vi "Main PXI4072.vi"() -> ()   [LabVIEW 2026]
uses:
  Drivers/PXI4072/Types/PXI4072 Settings.ctl
  <instrlib>/niDMM/nidmm.llb/niDMM Function.ctl
  <instrlib>/niDMM/nidmm.llb/niDMM Resolution in Digits.ctl
  App Types/Typedef/PXI4072 Runtime.ctl
  App Types/Typedef/PXI4072 Command Message.ctl
  App Types/Enums/PXI4072 Command.ctl
  App Types/Typedef/PXI4072 UI Update.ctl
  App Types/Enums/PXI4072 Instrument Triggered Events.ctl
  App Types/Enums/PXI4072 UI States.ctl
  App Types/References/PXI4072 All UI References.ctl
  App Types/References/PXI4072 Boolean UI References.ctl
  App Types/References/PXI4072 String UI References.ctl
  App Types/References/PXI4072 Numeric UI References.ctl
  App Types/References/PXI4072 Other UI Rerences.ctl
  Common/Types/Enum/Bench Modules.ctl
  <vilib>/event_ctls.llb/usereventprio.ctl
  App Types/Globals/PXI4072 UI Global Refs.vi
  UI/UI Manager/Actions/PXI4072 Set Refs.vi
  UI/UI Manager/Actions/PXI4072 Initialize.vi
  UI/UI Manager/Actions/PXI4072 Update UI Status.vi
  Drivers/PXI4072/PXI4072.lvlib
  Common/PXI_Common.lvlib
  Common/Types/Typedef/Log Message Levels.ctl
  Common/Types/Typedef/Log Message.ctl
panel:
  out "Measurement":dbl format="%.5f"
  in  "Measurement Settings":T1={"Function"=enum."DC Volts", "Resolution in Digits"=5.5, "Range"=10.0} {"Range" format="%.2f"; "Resolution in Digits" items=["3 1/2"=3.5, "4 1/2"=4.5, "5 1/2"=5.5, "6 1/2"=6.5, "7 1/2"=7.5]}
  in  "Apply Button":bool
  in  "Error":string
  out "Units":string
  in  "Reset Button":bool
  in  "Self Test Button":bool
  in  "Stop Button":bool
  in  "Continous Button":bool
  in  "Measure Button":bool
  in  "Status":string
  out "Connected?":bool
  in  "Disconnect Button":bool
  in  "Connect Button":bool
  in  "Resouce Name":refnum<k15> caption="Resource Name"
  out "error out":errorcluster
  in  "error in (no error)":errorcluster
  # "NI PXI-4072 DIGITAL MULTIMETER"
  # "MEASUREMENT SETUP"
  # "DEVICE"
  # "ACQUISITION"
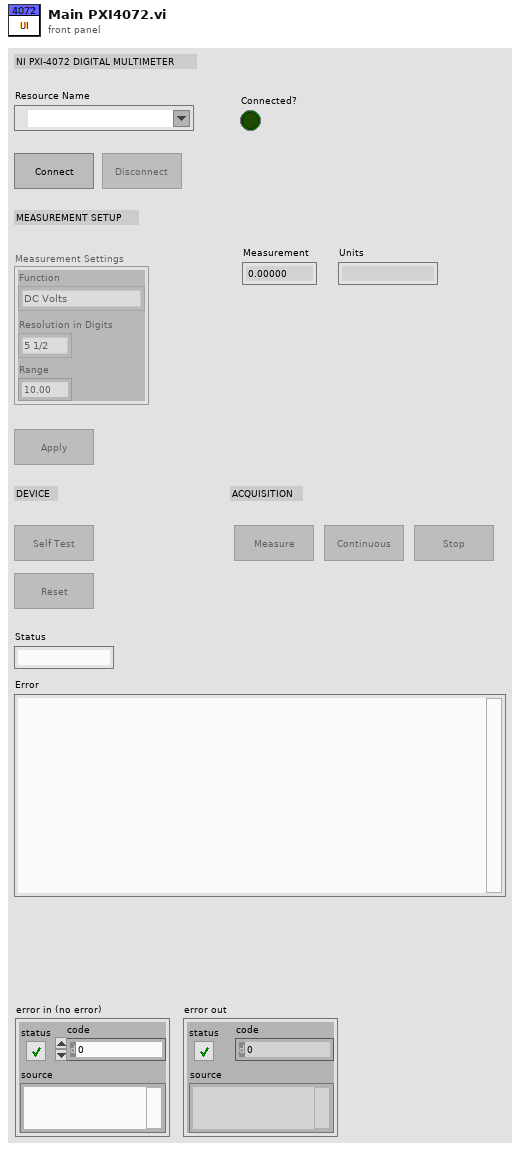
[diagram p1: front panel]
types:
  T1 = typedef "PXI4072.lvlib/PXI4072 Settings.ctl" = cluster{"Function":T2, "Resolution in Digits":T3, "Range":dbl}
  T2 = typedef "niDMM Function.ctl" = enum16{"DC Volts", "AC Volts", "DC Current", "AC Current", "2-wire Resistance", "4-wire Resistance", "Diode", "Frequency", "Period", "AC Volts DC Coupled", "Capacitance", "Inductance", "Temperature"}
  T3 = typedef "niDMM Resolution in Digits.ctl" = dbl
  T4 = typedef "PXI_Common.lvlib/Log Message.ctl" = cluster{"Timestamp":string, "Level":T5, "Instrument":T6, "Slot":string, "Code":i32, "Soruce":string, "Message":string}
  T5 = typedef "PXI_Common.lvlib/Log Message Levels.ctl" = enum16{"DEBUG", "INFO", "WARNING", "ERROR"}
  T6 = typedef "PXI_Common.lvlib/Bench Modules.ctl" = enum16{"Common", "PXI4072", "PXI6259", "PXI6224", "PXI4130", "PXI8431"}
  T7 = typedef "PXI4072 UI States.ctl" = enum16{"Get UI Refs", "UI Initialize", "Handle Events"}
  T8 = typedef "PXI4072 UI Update.ctl" = cluster{"Elements":cluster{"Event":T9, "Measurement":dbl, "Connected":bool, "Text":string, "Error":errorcluster}}
  T9 = typedef "PXI4072 Instrument Triggered Events.ctl" = enum16{"Measurement", "Connection", "Status", "Self Test", "Error"}
  T10 = typedef "PXI4072 Command Message.ctl" = cluster{"App Commands":T11, "Measurement Settings":T1}
  T11 = typedef "PXI4072 Command.ctl" = enum16{"Disconnect", "Initialize", "Configure", "Measure Single", "Reset", "Self Test", "Shutdown"}
  T12 = typedef "PXI4072 Runtime.ctl" = cluster{"Session Handle":refnum<k15>, "Measurement Settings":T1, "Connected":bool, "Last Measurement":dbl, "Last Error":errorcluster}
  T13 = typedef "PXI4072 All UI References.ctl" = cluster{"Boolean":T14, "String":T15, "Numeric":T16, "Other":T17}
  T14 = typedef "PXI4072 Boolean UI References.ctl" = cluster{"Connected?":refnum<vi>, "Reset Button":refnum<vi>, "Connect Button":refnum<vi>, "Apply Button":refnum<vi>, "Disconnect Button":refnum<vi>, "Measure Button":refnum<vi>, "Self Test Button":refnum<vi>, "Continous Button":refnum<vi>, "Stop Button":refnum<vi>}
  T15 = typedef "PXI4072 String UI References.ctl" = cluster{"Status":refnum<vi>, "Units":refnum<vi>, "Error":refnum<vi>}
  T16 = typedef "PXI4072 Numeric UI References.ctl" = cluster{"Measurement":refnum<vi>}
  T17 = typedef "PXI4072 Other UI Rerences.ctl" = cluster{"Resouce Name":refnum<vi>, "Measurement Settings":refnum<vi>}
  T18 = cluster{"Event":T9, "Measurement":dbl, "Connected":bool, "Text":string, "Error":errorcluster}
  T19 = typedef "usereventprio.ctl" = enum32{"high priority", "normal priority"}
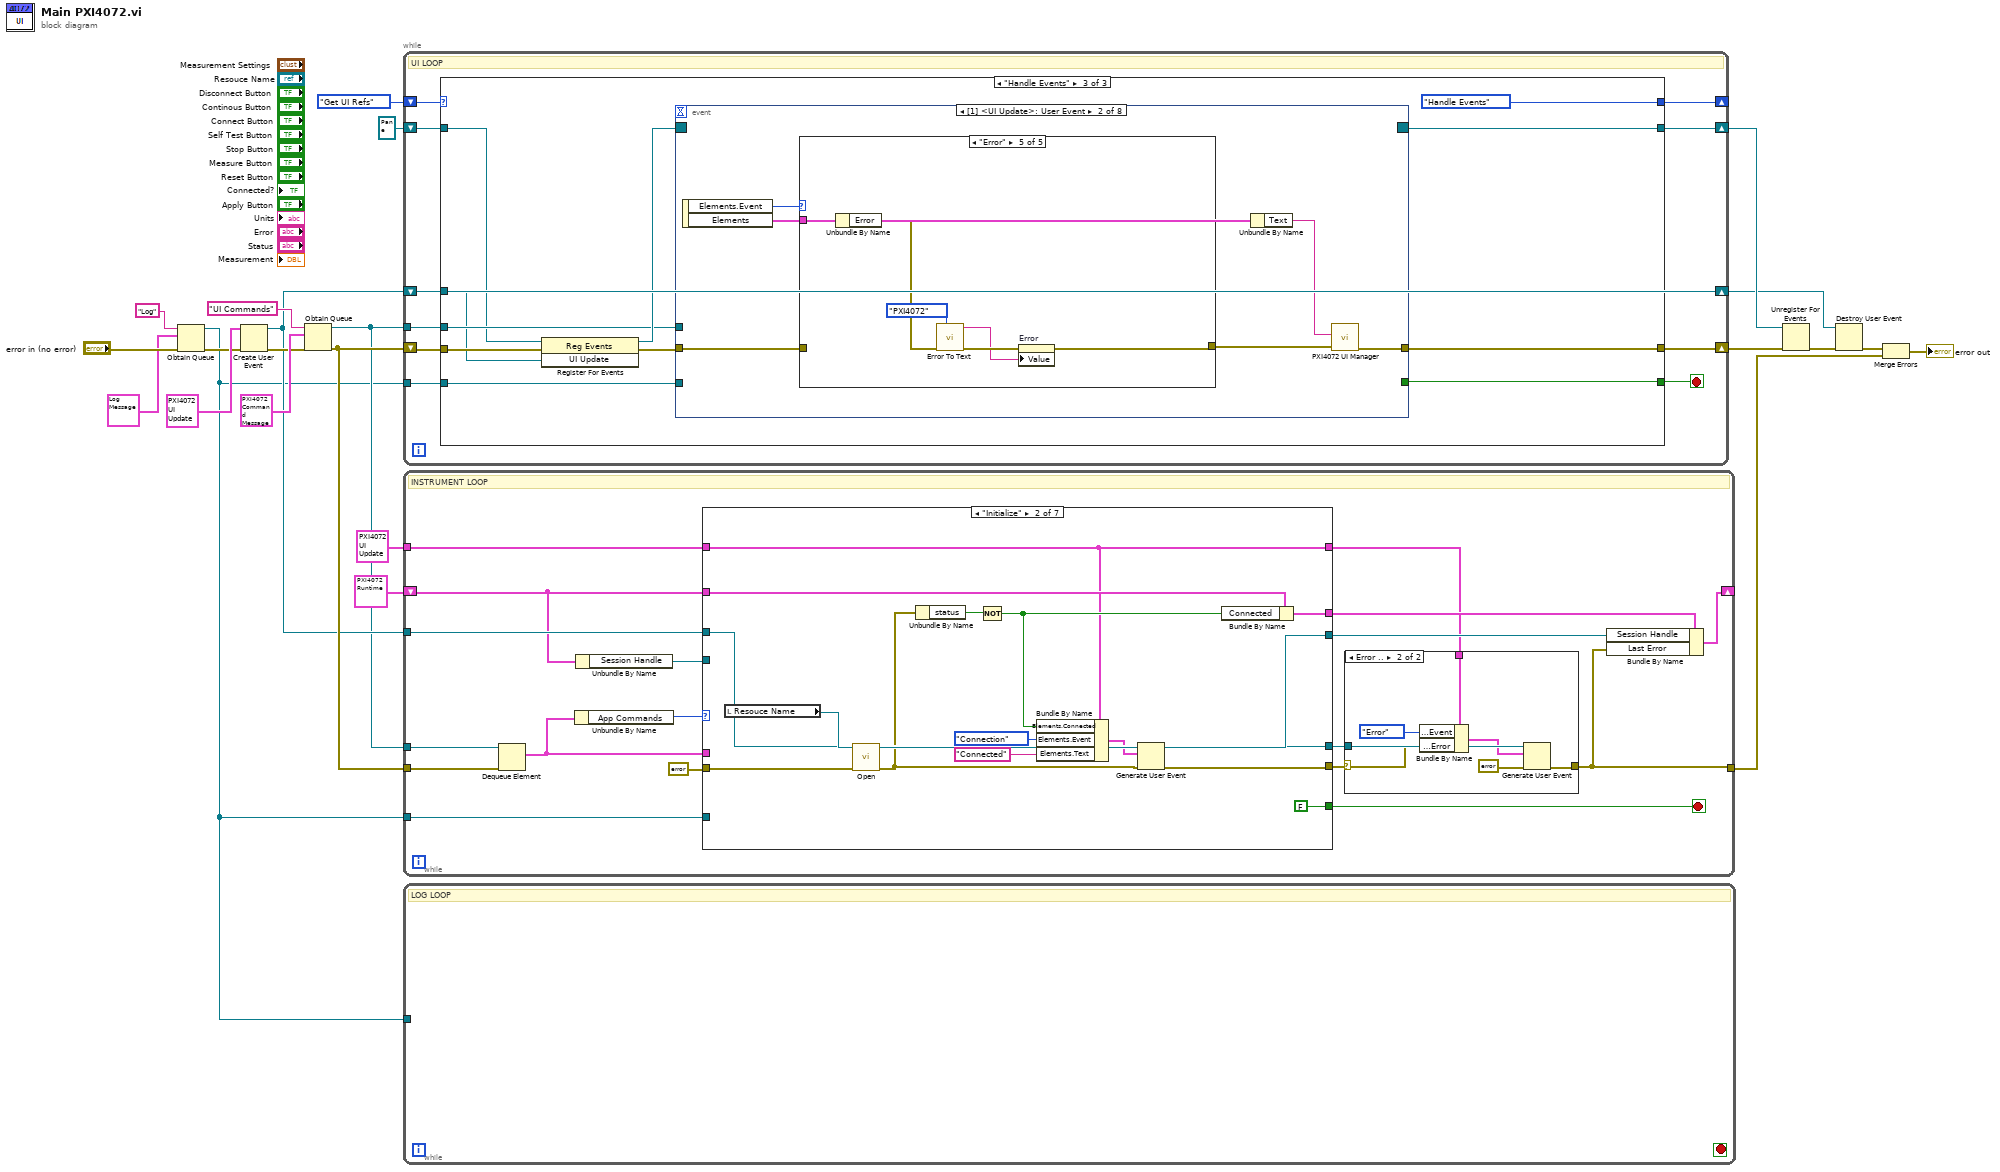
[diagram p0: block diagram]
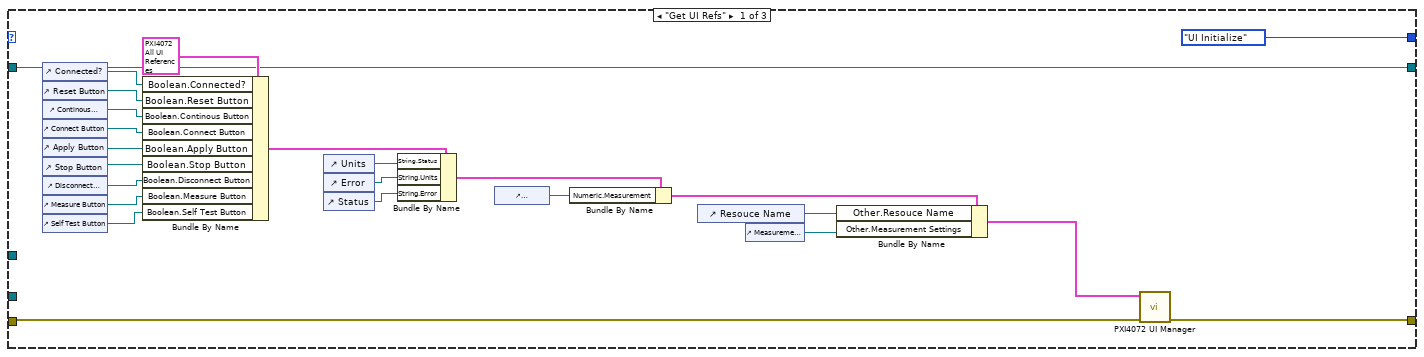
[diagram p2: hidden frame]
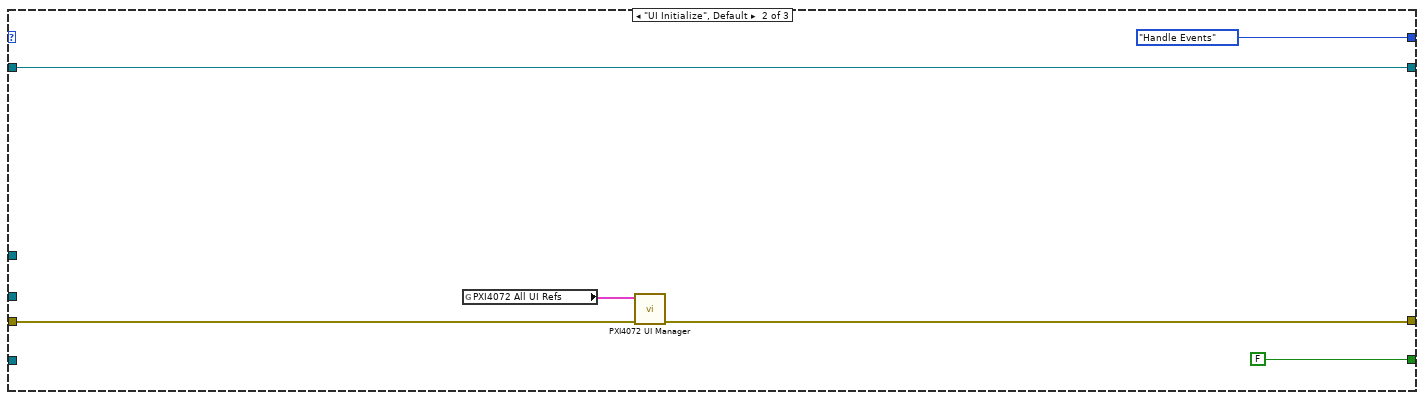
[diagram p3: hidden frame]
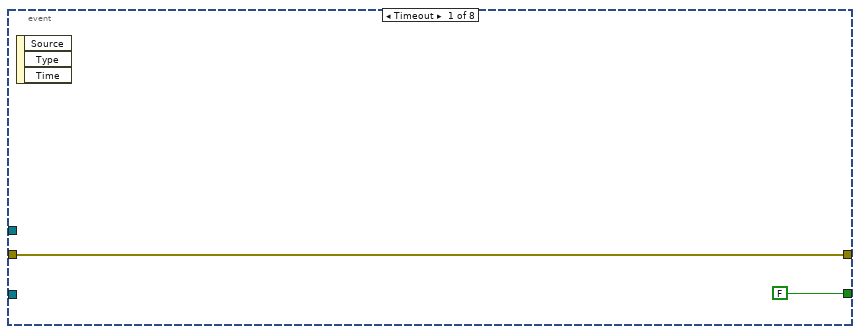
[diagram p4: hidden frame]
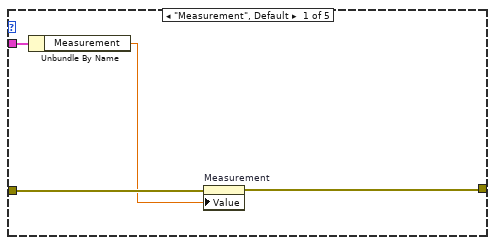
[diagram p5: hidden frame]
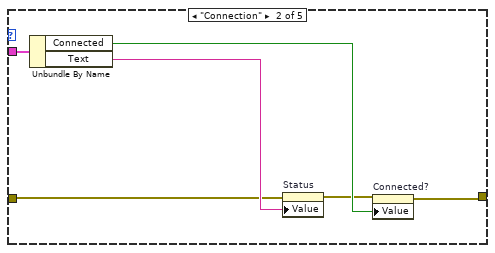
[diagram p6: hidden frame]
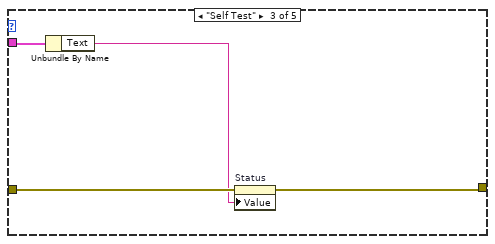
[diagram p7: hidden frame]
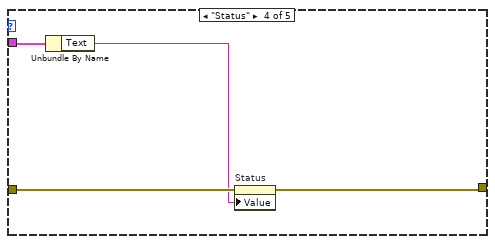
[diagram p8: hidden frame]
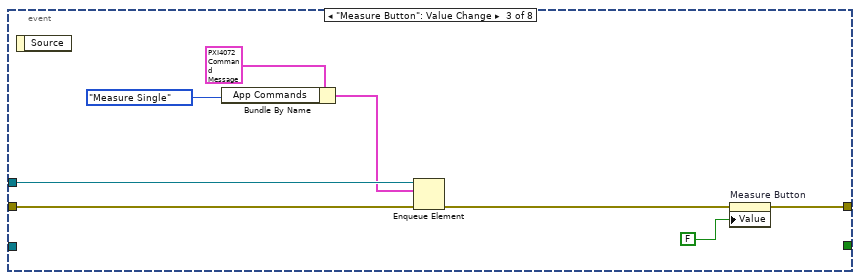
[diagram p9: hidden frame]
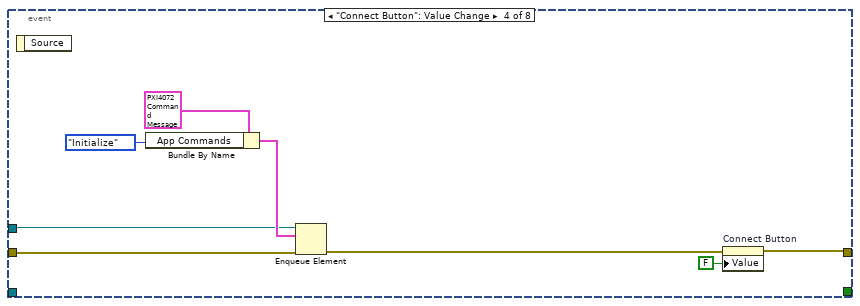
[diagram p10: hidden frame]
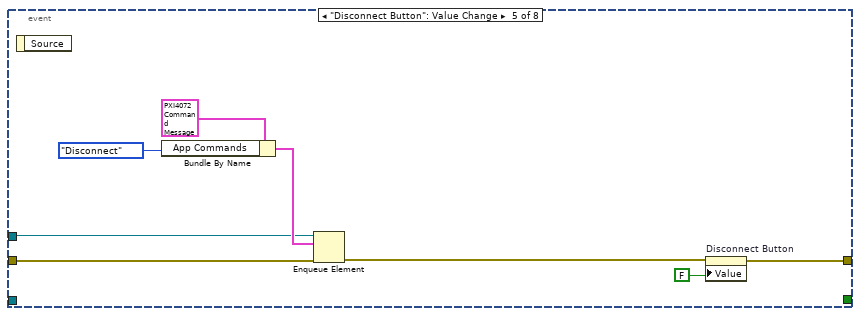
[diagram p11: hidden frame]
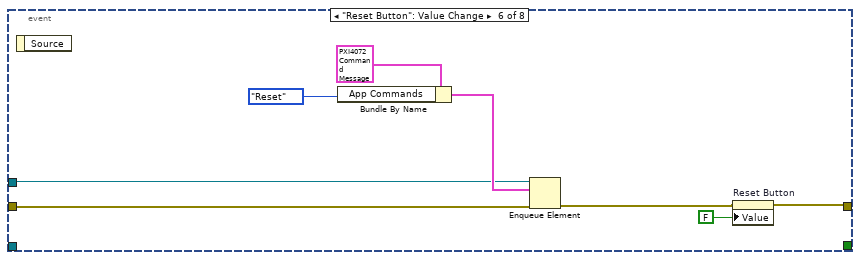
[diagram p12: hidden frame]
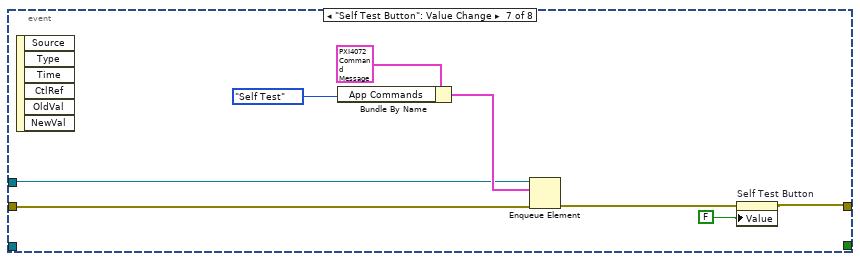
[diagram p13: hidden frame]
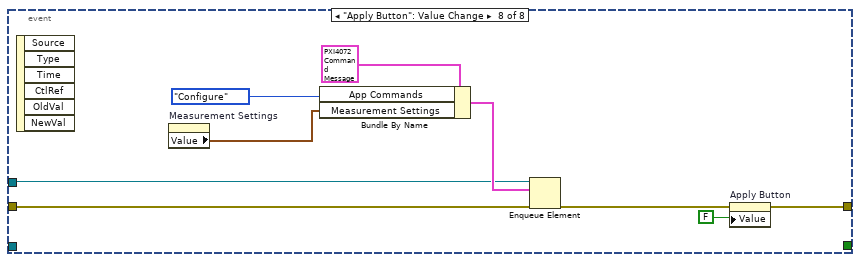
[diagram p14: hidden frame]
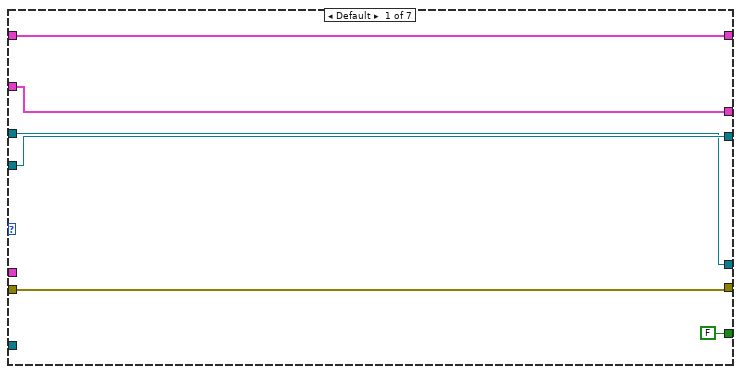
[diagram p16: hidden frame]
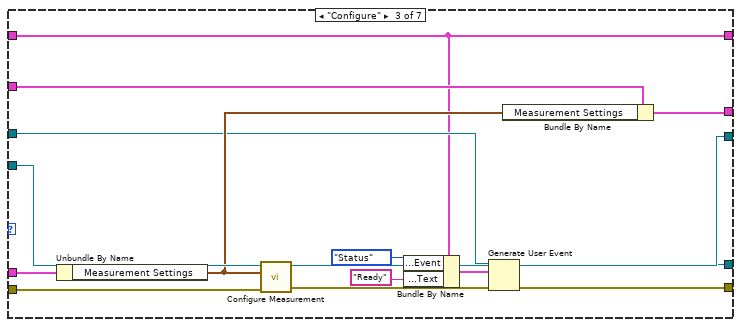
[diagram p17: hidden frame]
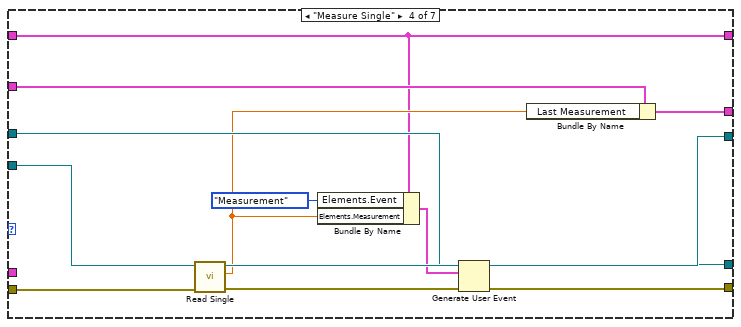
[diagram p18: hidden frame]
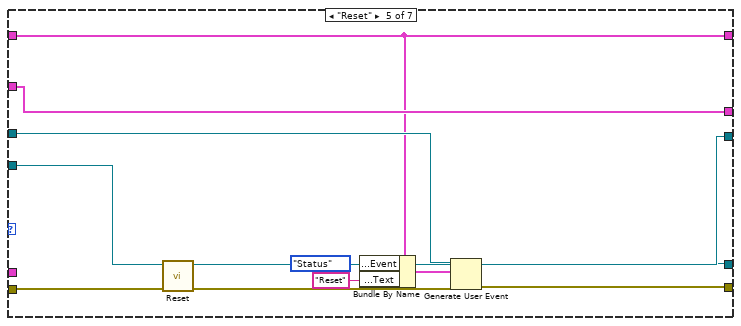
[diagram p19: hidden frame]
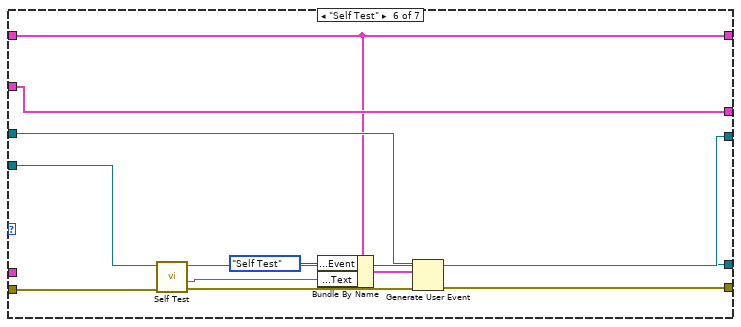
[diagram p20: hidden frame]
diagram:
  n1 = Obtain Queue(name (unnamed)="Log", element data type=T4 {"Timestamp"="", "Level"=enum."DEBUG", "Instrument"=enum."Common", "Slot"="", "Code"=0, "Soruce"="", "Message"=""} ("Log Message"), error in (no error)="error in (no error)") -> (queue out=w1:refnum<queue>, error out=w4:errorcluster)  [unwired: 2 in, 1 out]
  n2 = Create User Event(user event datatype=T8 {"Elements"={"Event"=enum."Measurement", "Measurement"=0.0, "Connected"=FALSE, "Text"="", "Error"={"status"=FALSE, "code"=0, "source"=""}}} ("UI Update"), error in=w4) -> (user event=w15:refnum<user-event>, error out=w17:errorcluster)
  n3 = Obtain Queue(name (unnamed)="UI Commands", element data type=T10 {"App Commands"=enum."Initialize", "Measurement Settings"={"Function"=enum."DC Volts", "Resolution in Digits"=5.5, "Range"=10.0}} ("Command Message"), error in (no error)=w17) -> (queue out=w7:refnum<queue>, error out=w21:errorcluster)  [unwired: 2 in, 1 out]
  n4 = while {
    tunnel: w7 -> [w29]
    shift-right: [w33] -> w14
    shift-left: w21 -> [w31]
    shift-right: [w27] -> _
    shift-left: PXI4072_UI_States."Get UI Refs" ("Enum") -> [w28]
    shift-right: [w26] -> w10
    shift-left: w15 -> [w26]
    shift-right: [w30] -> w13
    shift-left: refnum<event-registration> refnum ("event registration refnum") -> [w25]
    tunnel: w1 -> [w24]
    stop <- w32 stop-if-true
    # "UI LOOP"
    n5 = case shown="\"Handle Events\"" w28 {
      tunnel: [w38 w60 w74] -> w33
      tunnel: [_ FALSE w73] -> w32
      tunnel: w31 -> [w37 w61 w72]
      tunnel: [w34 w58 w69] -> w30
      tunnel: w26 -> [_ _ w66]
      tunnel: w29 -> [_ _ w68]
      tunnel: [PXI4072_UI_States."UI Initialize" ("Enum") PXI4072_UI_States."Handle Events" ("Enum") PXI4072_UI_States."Handle Events" ("Enum")] -> w27
      tunnel: w25 -> [w34 w58 w65]
      tunnel: w24 -> [_ _ w64]
      frame "Get UI Refs" {
        n6 = control-ref of="Connected?"() -> (w56:refnum<vi>)
        n7 = control-ref of="Reset Button"() -> (w55:refnum<vi>)
        n8 = control-ref of="Continous Button"() -> (w54:refnum<vi>)
        n9 = control-ref of="Connect Button"() -> (w53:refnum<vi>)
        n10 = control-ref of="Apply Button"() -> (w52:refnum<vi>)
        n11 = control-ref of="Stop Button"() -> (w51:refnum<vi>)
        n12 = control-ref of="Disconnect Button"() -> (w50:refnum<vi>)
        n13 = control-ref of="Measure Button"() -> (w49:refnum<vi>)
        n14 = control-ref of="Self Test Button"() -> (w48:refnum<vi>)
        n15 = Bundle By Name(cluster=T13 {"Boolean"={"Connected?"=refnum, "Reset Button"=refnum, "Connect Button"=refnum, "Apply Button"=refnum, "Disconnect Button"=refnum, "Measure Button"=refnum, "Self Test Button"=refnum, "Continous Button"=refnum, "Stop Button"=refnum}, "String"={"Status"=refnum, "Units"=refnum, "Error"=refnum}, "Numeric"={"Measurement"=refnum}, "Other"={"Resouce Name"=refnum, "Measurement Settings"=refnum}} ("PXI4072 All UI Refs"), "Boolean.Connected?"=w56, "Boolean.Reset Button"=w55, "Boolean.Continous Button"=w54, "Boolean.Connect Button"=w53, "Boolean.Apply Button"=w52, "Boolean.Stop Button"=w51, "Boolean.Disconnect Button"=w50, "Boolean.Measure Button"=w49, "Boolean.Self Test Button"=w48) -> (w47:T13)
        n16 = control-ref of="Units"() -> (w46:refnum<vi>)
        n17 = control-ref of="Error"() -> (w45:refnum<vi>)
        n18 = control-ref of="Status"() -> (w44:refnum<vi>)
        n19 = Bundle By Name(cluster=w47, "String.Status"=w46, "String.Units"=w45, "String.Error"=w44) -> (w43:T13)
        n20 = control-ref of="Measurement"() -> (w42:refnum<vi>)
        n21 = Bundle By Name(cluster=w43, "Numeric.Measurement"=w42) -> (w41:T13)
        n22 = control-ref of="Resouce Name"() -> (w40:refnum<vi>)
        n23 = control-ref of="Measurement Settings"() -> (w39:refnum<vi>)
        n24 = Bundle By Name(cluster=w41, "Other.Resouce Name"=w40, "Other.Measurement Settings"=w39) -> (w36:T13)
        n25 = call-poly "PXI4072 UI Manager.vi"("error in (no error)"=w37, "PXI4072 All UI Refs"=w36) -> ("error out"=w38:errorcluster)  [unwired: 9 in]
      }
      frame "UI Initialize", Default {
        n26 = global read "PXI4072 UI Global Refs.vi" "PXI4072 All UI Refs"() -> (w59:T13)
        n27 = call-poly "PXI4072 UI Manager.vi"("error in (no error)"=w61, "PXI4072 All UI Refs"=w59) -> ("error out"=w60:errorcluster)  [unwired: 9 in]
      }
      frame "Handle Events" {
        n28 = register-events(reference=w65, error in=w72, w66) -> (reference out=w70:refnum<event-registration>, error out=w71:errorcluster)
        n29 = event shown="[1] <UI Update>: User Event" {
          selector: w70 -> [_ _ _ _ _ _ _ _]
          dyn-events: [_ _ _ _ _ _ _ _] -> w69
          timeout: _ -> [_ _ _ _ _ _ _ _]
          tunnel: w71 -> [w76 w81 w112 w118 w128 w136 w144 w153]
          tunnel: [w76 w79 w114 w122 w125 w133 w141 w149] -> w74
          tunnel: [FALSE _ _ _ _ _ _ _] -> w73
          tunnel: w68 -> [_ _ w111 w115 w126 w134 w142 w151]
          tunnel: w64 -> [_ _ _ _ _ _ _ _]
          event Timeout {
            n30 = event-data() -> ()  [unwired: 1 in, 3 out]
          }
          event User Event {
            n31 = event-data() -> ("Elements.Event"=w82:T9, "Elements"=w78:T18)  [unwired: 1 in]
            n32 = case shown="\"Error\"" w82 {
              tunnel: w81 -> [w86 w87 w95 w99 _]
              tunnel: [w85 w91 w94 w98 w105] -> w80
              tunnel: w78 -> [w84 w92 w96 w100 w106]
              frame "Measurement", Default {
                n33 = Unbundle By Name(w84) -> ("Measurement"=w83:dbl)
                n34 = property on="Measurement" class="DigNum (strict)"(error in=w86, "Value"=w83) -> (error out=w85:errorcluster)  [unwired: 1 in, 1 out]
              }
              frame "Connection" {
                n35 = Unbundle By Name(w92) -> ("Connected"=w90:bool, "Text"=w88:string)
                n36 = property on="Status" class="Str"(error in=w87, "Value"=w88) -> (error out=w89:errorcluster)  [unwired: 1 in, 1 out]
                n37 = property on="Connected?" class="Bool (strict)"(error in=w89, "Value"=w90) -> (error out=w91:errorcluster)  [unwired: 1 in, 1 out]
              }
              frame "Self Test" {
                n38 = Unbundle By Name(w96) -> ("Text"=w93:string)
                n39 = property on="Status" class="Str"(error in=w95, "Value"=w93) -> (error out=w94:errorcluster)  [unwired: 1 in, 1 out]
              }
              frame "Status" {
                n40 = Unbundle By Name(w100) -> ("Text"=w97:string)
                n41 = property on="Status" class="Str"(error in=w99, "Value"=w97) -> (error out=w98:errorcluster)  [unwired: 1 in, 1 out]
              }
              frame "Error" {
                n42 = Unbundle By Name(w106) -> ("Error"=w103:errorcluster)
                n43 = call "Error To Text.vi"("Bench Module"=Bench_Modules."PXI4072", "error in (no error)"=w103) -> ("error out"=w104:errorcluster, "message"=w102:string)  [unwired: 8 in]
                n44 = property on="Error" class="Str"(error in=w104, "Value"=w102) -> (error out=w105:errorcluster)  [unwired: 1 in, 1 out]
              }
            }
            n45 = Unbundle By Name(w78) -> ("Text"=w77:string)
            n46 = call-poly "PXI4072 UI Manager.vi"("error in (no error)"=w80, "Instr Status"=w77) -> ("error out"=w79:errorcluster)  [unwired: 9 in]
          }
          event "Measure Button": Value Change {
            n47 = event-data() -> ()  [unwired: 1 in, 1 out]
            n48 = Bundle By Name(cluster=T10 {"App Commands"=enum."Initialize", "Measurement Settings"={"Function"=enum."DC Volts", "Resolution in Digits"=5.5, "Range"=10.0}} ("element"), "App Commands"=PXI4072_Command."Measure Single") -> (w108:T10)
            n49 = Enqueue Element(queue=w111, element=w108, error in (no error)=w112) -> (error out=w110:errorcluster)  [unwired: 1 in, 2 out]
            n50 = property on="Measure Button" class="Bool (strict)"(error in=w110, "Value"=FALSE ("Measure Button")) -> (error out=w114:errorcluster)  [unwired: 1 in, 1 out]
          }
          event "Connect Button": Value Change {
            n51 = event-data() -> ()  [unwired: 1 in, 1 out]
            n52 = Bundle By Name(cluster=T10 {"App Commands"=enum."Initialize", "Measurement Settings"={"Function"=enum."DC Volts", "Resolution in Digits"=5.5, "Range"=10.0}} ("element"), "App Commands"=PXI4072_Command."Initialize") -> (w119:T10)
            n53 = Enqueue Element(queue=w115, element=w119, error in (no error)=w118) -> (error out=w117:errorcluster)  [unwired: 1 in, 2 out]
            n54 = property on="Connect Button" class="Bool (strict)"(error in=w117, "Value"=FALSE ("Connect Button")) -> (error out=w122:errorcluster)  [unwired: 1 in, 1 out]
          }
          event "Disconnect Button": Value Change {
            n55 = event-data() -> ()  [unwired: 1 in, 1 out]
            n56 = Bundle By Name(cluster=T10 {"App Commands"=enum."Initialize", "Measurement Settings"={"Function"=enum."DC Volts", "Resolution in Digits"=5.5, "Range"=10.0}} ("element"), "App Commands"=PXI4072_Command."Disconnect") -> (w129:T10)
            n57 = Enqueue Element(queue=w126, element=w129, error in (no error)=w128) -> (error out=w123:errorcluster)  [unwired: 1 in, 2 out]
            n58 = property on="Disconnect Button" class="Bool (strict)"(error in=w123, "Value"=FALSE ("Connect Button")) -> (error out=w125:errorcluster)  [unwired: 1 in, 1 out]
          }
          event "Reset Button": Value Change {
            n59 = event-data() -> ()  [unwired: 1 in, 1 out]
            n60 = Bundle By Name(cluster=T10 {"App Commands"=enum."Initialize", "Measurement Settings"={"Function"=enum."DC Volts", "Resolution in Digits"=5.5, "Range"=10.0}} ("element"), "App Commands"=PXI4072_Command."Reset") -> (w137:T10)
            n61 = Enqueue Element(queue=w134, element=w137, error in (no error)=w136) -> (error out=w132:errorcluster)  [unwired: 1 in, 2 out]
            n62 = property on="Reset Button" class="Bool (strict)"(error in=w132, "Value"=FALSE ("Connect Button")) -> (error out=w133:errorcluster)  [unwired: 1 in, 1 out]
          }
          event "Self Test Button": Value Change {
            n63 = event-data() -> ()  [unwired: 1 in, 6 out]
            n64 = Bundle By Name(cluster=T10 {"App Commands"=enum."Initialize", "Measurement Settings"={"Function"=enum."DC Volts", "Resolution in Digits"=5.5, "Range"=10.0}} ("element"), "App Commands"=PXI4072_Command."Self Test") -> (w145:T10)
            n65 = Enqueue Element(queue=w142, element=w145, error in (no error)=w144) -> (error out=w140:errorcluster)  [unwired: 1 in, 2 out]
            n66 = property on="Self Test Button" class="Bool (strict)"(error in=w140, "Value"=FALSE ("Connect Button")) -> (error out=w141:errorcluster)  [unwired: 1 in, 1 out]
          }
          event "Apply Button": Value Change {
            n67 = event-data() -> ()  [unwired: 1 in, 6 out]
            n68 = property on="Measurement Settings" class="Clust (strict)"() -> ("Value"=w150:T1)  [unwired: 2 in, 2 out]
            n69 = Bundle By Name(cluster=T10 {"App Commands"=enum."Initialize", "Measurement Settings"={"Function"=enum."DC Volts", "Resolution in Digits"=5.5, "Range"=10.0}} ("element"), "App Commands"=PXI4072_Command."Configure", "Measurement Settings"=w150) -> (w154:T10)
            n70 = Enqueue Element(queue=w151, element=w154, error in (no error)=w153) -> (error out=w148:errorcluster)  [unwired: 1 in, 2 out]
            n71 = property on="Apply Button" class="Bool (strict)"(error in=w148, "Value"=FALSE ("Connect Button")) -> (error out=w149:errorcluster)  [unwired: 1 in, 1 out]
          }
        }
      }
    }
  }
  n72 = while {
    tunnel: w7 -> [w173]
    shift-right: [w170] -> _
    shift-left: T12 {"Session Handle"="", "Measurement Settings"={"Function"=enum."DC Volts", "Resolution in Digits"=5.5, "Range"=10.0}, "Connected"=FALSE, "Last Measurement"=0.0, "Last Error"={"status"=FALSE, "code"=0, "source"=""}} ("Runtime Data") -> [w167]
    tunnel: w15 -> [w168]
    tunnel: T8 {"Elements"={"Event"=enum."Measurement", "Measurement"=0.0, "Connected"=FALSE, "Text"="", "Error"={"status"=FALSE, "code"=0, "source"=""}}} ("event data") -> [w165]
    tunnel: w21 -> [w166]
    tunnel: [w159] -> w18
    tunnel: w1 -> [w156]
    stop <- w169 stop-if-true
    # "INSTRUMENT LOOP"
    n73 = Dequeue Element(queue=w173, error in (no error)=w166) -> (element=w164:T10)  [unwired: 1 in, 3 out]
    n74 = Unbundle By Name(w164) -> ("App Commands"=w163:T11)
    n75 = Unbundle By Name(w167) -> ("Session Handle"=w162:refnum<k15>)
    n76 = case shown="\"Initialize\"" w163 {
      tunnel: errorcluster {"status"=FALSE, "code"=0, "source"=""} ("no error constant") -> [w187 w203 w218 w231 w243 w255 w265]
      tunnel: [w187 w196 w210 w225 w238 w244 w264] -> w160
      tunnel: w167 -> [w185 w202 w214 w228 w240 w248 w263]
      tunnel: [w185 w201 w213 w227 w240 w248 w263] -> w172
      tunnel: [w186 w199 w216 w229 w241 w253 w258] -> w171
      tunnel: w162 -> [w186 _ w217 w230 w242 w254 w259]
      tunnel: w164 -> [_ _ w215 _ _ _ _]
      tunnel: [FALSE FALSE _ _ _ _ _] -> w169
      tunnel: w168 -> [w183 w195 w209 w224 w237 w249 w261]
      tunnel: w165 -> [w182 w189 w205 w219 w233 w246 w260]
      tunnel: [w182 w189 w205 w219 w233 w246 w257] -> w157
      tunnel: [w183 w188 w204 w220 w232 w245 w256] -> w158
      tunnel: w156 -> [_ _ _ _ _ _ _]
      frame Default {
      }
      frame "Initialize" {
        n77 = local read "Resouce Name"() -> (w200:refnum<k15>)
        n78 = call "Open.vi"("error in (no error)"=w203, "Resouce Name"=w200) -> ("error out"=w192:errorcluster, "Session Handle Out"=w199:refnum<k15>)  [unwired: 8 in]
        n79 = Unbundle By Name(w192) -> ("status"=w198:bool)
        n80 = Not(x=w198) -> (.not. x?=w193:bool)
        n81 = Bundle By Name(cluster=w189, "Elements.Connected"=w193, "Elements.Event"=PXI4072_Instrument_Triggered_Events."Connection", "Elements.Text"="Connected") -> (w194:T8)
        n82 = Generate User Event(user event=w195, event data cluster=w194, error in=w192) -> (user event out=w188:refnum<user-event>, error out=w196:errorcluster)  [unwired: 1 in]
        n83 = Bundle By Name(cluster=w202, "Connected"=w193) -> (w201:T12)
      }
      frame "Configure" {
        n84 = Unbundle By Name(w215) -> ("Measurement Settings"=w212:T1)
        n85 = call "Configure Measurement.vi"("error in (no error)"=w218, "Measurement Settings"=w212, "Session Handle"=w217) -> ("error out"=w211:errorcluster, "Session Handle Out"=w216:refnum<k15>)  [unwired: 7 in]
        n86 = Bundle By Name(cluster=w205, "Elements.Event"=PXI4072_Instrument_Triggered_Events."Status", "Elements.Text"="Ready") -> (w208:T8)
        n87 = Generate User Event(user event=w209, event data cluster=w208, error in=w211) -> (user event out=w204:refnum<user-event>, error out=w210:errorcluster)  [unwired: 1 in]
        n88 = Bundle By Name(cluster=w214, "Measurement Settings"=w212) -> (w213:T12)
      }
      frame "Measure Single" {
        n89 = call "Read Single.vi"("error in (no error)"=w231, "Session Handle"=w230) -> ("error out"=w226:errorcluster, "Measurement"=w222:dbl, "instrument handle out"=w229:refnum<k15>)  [unwired: 7 in]
        n90 = Bundle By Name(cluster=w219, "Elements.Event"=PXI4072_Instrument_Triggered_Events."Measurement", "Elements.Measurement"=w222) -> (w223:T8)
        n91 = Generate User Event(user event=w224, event data cluster=w223, error in=w226) -> (user event out=w220:refnum<user-event>, error out=w225:errorcluster)  [unwired: 1 in]
        n92 = Bundle By Name(cluster=w228, "Last Measurement"=w222) -> (w227:T12)
      }
      frame "Reset" {
        n93 = call "Reset.vi"("error in (no error)"=w243, "Session Handle"=w242) -> ("error out"=w239:errorcluster, "Session Handle Out"=w241:refnum<k15>)  [unwired: 8 in]
        n94 = Bundle By Name(cluster=w233, "Elements.Event"=PXI4072_Instrument_Triggered_Events."Status", "Elements.Text"="Reset") -> (w236:T8)
        n95 = Generate User Event(user event=w237, event data cluster=w236, error in=w239) -> (user event out=w232:refnum<user-event>, error out=w238:errorcluster)  [unwired: 1 in]
      }
      frame "Self Test" {
        n96 = call "Self Test.vi"("error in (no error)"=w255, "Session Handle"=w254) -> ("error out"=w252:errorcluster, "Self Test Message"=w251:string, "Session Handle Out"=w253:refnum<k15>)  [unwired: 6 in, 1 out]
        n97 = Bundle By Name(cluster=w246, "Elements.Event"=PXI4072_Instrument_Triggered_Events."Self Test", "Elements.Text"=w251) -> (w250:T8)
        n98 = Generate User Event(user event=w249, event data cluster=w250, error in=w252) -> (user event out=w245:refnum<user-event>, error out=w244:errorcluster)  [unwired: 1 in]
      }
      frame "Disconnect" {
        n99 = Unbundle By Name(w263) -> ("Connected"=w262:bool)
        n100 = case shown="False" w262 {
          tunnel: w265 -> [w269 w281]
          tunnel: [w269 w280] -> w264
          tunnel: w259 -> [w268 w274]
          tunnel: w261 -> [w266 w279]
          tunnel: w260 -> [w267 w271]
          tunnel: [w268 w274] -> w258
          tunnel: [w267 w271] -> w257
          tunnel: [w266 w270] -> w256
          frame False {
          }
          frame True {
            n101 = call "Close.vi"("error in (no error)"=w281, "Session Handle"=w274) -> ("error out"=w276:errorcluster)  [unwired: 9 in]
            n102 = Bundle By Name(cluster=w271, "Elements.Event"=PXI4072_Instrument_Triggered_Events."Connection", "Elements.Connected"=FALSE, "Elements.Text"="Disconnected") -> (w278:T8)
            n103 = Generate User Event(priority (normal)=usereventprio."high priority", user event=w279, event data cluster=w278, error in=w276) -> (user event out=w270:refnum<user-event>, error out=w280:errorcluster)
          }
        }
      }
    }
    n104 = case shown="Error .." w160 {
      selector: w160 -> [w174 w178]
      tunnel: [w174 w180] -> w159
      tunnel: w158 -> [_ w181]
      tunnel: w157 -> [_ w177]
      frame No Error {
      }
      frame Error {
        n105 = Bundle By Name(cluster=w177, "Elements.Event"=PXI4072_Instrument_Triggered_Events."Error", "Elements.Error"=w178) -> (w175:T8)
        n106 = Generate User Event(user event=w181, event data cluster=w175, error in=errorcluster {"status"=FALSE, "code"=0, "source"=""} ("no error constant")) -> (error out=w180:errorcluster)  [unwired: 1 in, 1 out]
      }
    }
    n107 = Bundle By Name(cluster=w172, "Session Handle"=w171, "Last Error"=w159) -> (w170:T12)
  }
  n108 = while {
    tunnel: w1 -> [_]
    stop <- _ stop-if-true
    # "LOG LOOP"
  }
  n109 = Unregister For Events(event registration refnum=w13, error in=w14) -> (error out=w12:errorcluster)
  n110 = Destroy User Event(user event=w10, error in=w12) -> (error out=w11:errorcluster)
  n111 = Merge Errors(w11, w18) -> (→"error out":errorcluster)
